vi "multiclamp_switchClamps_v02.vi"(8 "error in":i32, 9 "error in (no error)":errorcluster, 10 "which clamp":enum16{"VClamp", "IClamp"}(ring), 11 "Multiclamp Handle in":u32) -> (1 "error out":errorcluster, 2 "current clamp mode":enum16{"VClamp", "IClamp"}(ring))   [LabVIEW 2019]
uses:
  patcherBot_software_all/patcherBot_Software/patcherBot/AxMultiClampMsg.dll
panel:
  # "switch multiclamp mode (IClamp, VClamp)"
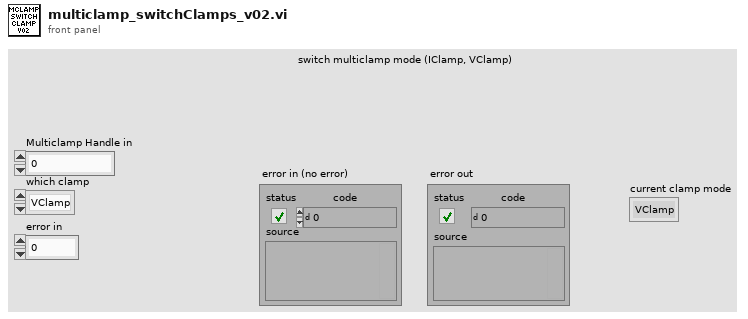
[diagram p1: front panel]
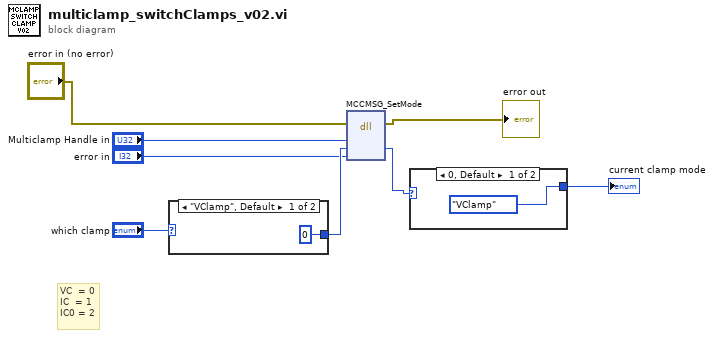
[diagram p0: block diagram]
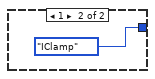
[diagram p2: hidden frame]
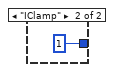
[diagram p3: hidden frame]
diagram:
  # "VC  = 0\nIC  = 1\nIC0 = 2"
  n1 = case shown="\"VClamp\", Default" "which clamp" {
    tunnel: [u32 0 u32 1] -> w7
    frame "VClamp", Default {
    }
    frame "IClamp" {
    }
  }
  n2 = dll-call lib="C:/Users/might/Dropbox (GaTech)/patcherBot_software_all/patcherBot_Software/patcherBot/AxMultiClampMsg.dll" fn="MCCMSG_SetMode"(error in="error in (no error)", "handle"="Multiclamp Handle in", "ModeConstant"=w7, "error"="error in") -> (error out=→"error out":errorcluster, "ModeConstant"=w2:u32)  [unwired: 5 in, 1 out]
  n3 = case shown="0, Default" w2 {
    tunnel: [enum16{"VClamp", "IClamp"}."VClamp" ("which clamp") enum16{"VClamp", "IClamp"}."IClamp" ("which clamp")] -> w1
    frame 0, Default {
    }
    frame 1 {
    }
  }
  "current clamp mode" <- w1
